vi "TARGET_856.vi"() -> ()   [LabVIEW 2018]
uses:
  <vilib>/Platform/TimedLoop/XDataNode/timing_clust.ctl
  <vilib>/Platform/TimedLoop/XDataNode/nitl_modes.ctl
  <vilib>/Platform/TimedLoop/XDataNode/wakeup.ctl
  <vilib>/rvi/eio/common/nirviEmuTemplateMethod_errors.vi
  <vilib>/rvi/Emulation/niFpgaGetClockAttributes.vi
  <vilib>/rvi/Emulation/niFpgaSctlEmulationGetInTimedLoop.vi
  <vilib>/rvi/Emulation/niFpgaEmulationReportErrorSimple.vi
  <vilib>/rvi/Emulation/niFpgaProcessEmulError.vi
  <vilib>/rvi/Emulation/niFpgaCriticalErrorInLSC.vi
  <vilib>/rvi/interface/RandomDataEmulation/niFpgaRandomDataHandleErrors.vi
  <vilib>/eio/EIONode/EIONode.xnode
  <vilib>/Platform/TimedLoop/XDataNode/XDataNode.xnode
  <vilib>/rvi/DataTransferAndStorage/Container/XNode/niFpgaContainer.xnode
  <vilib>/rvi/interface/RandomDataEmulation/nirviRandomDataFpgaReadWriteTemplate.vi
  <vilib>/Platform/TimedLoop/XDataNode/XDNodeRunTimeDep.lvlib
panel:
  out "READ":bool[](array[boolean])
  in  "Write Data":bool[](array[boolean])=[FALSE, FALSE, FALSE, FALSE, FALSE, FALSE, FALSE, FALSE, FALSE]
  in  "Enum":T1(ring)=enum."GREEN OFF"
  in  "Read(T)/Write(F)":bool
  in  "Command array":bool[](array[boolean])=[FALSE, FALSE, FALSE, FALSE, FALSE, FALSE, FALSE, FALSE, FALSE, FALSE, FALSE, FALSE, FALSE, FALSE, FALSE, FALSE, FALSE]
  in  "Конфигурация":bool
  in  "Остановка основного цикла":bool
  in  "Линейки":bool
  in  "Между кадрами":u8=1 caption="Между кадрами, мс"
  out "Элем.":u32
  out "Данные":u8
  in  "Направление бит":bool
  in  "CDS1_1":u8=2
  in  "CDS1_2":u8=4
  in  "CDS2_1":u8=5
  in  "CDS2_2":u8=7
  in  "ADC_1":u8=2
  in  "ADC_2":u8=7
  in  "RG_1":u8=1
  in  "RG_2":u8=2
  in  "PH21_1":u8=1
  in  "PH21_2":u8=6
  in  "PH11_1":u8=1
  in  "PH11_2":u8=6
  in  "HOR":u16=880
  in  "10":u8=10
  in  "LOW":u8=1
  in  "HIGH":u8=9
  in  "2017":u16=2017
  in  "PS1_2":u16=1809
  in  "PS1_1":u16=715
  in  "PS2_2":u16=1151
  in  "PS2_1":u16=496
  in  "PS3_2":u16=1589
  in  "PS3_1":u16=934
  in  "PS4_2":u16=1371
  in  "PS4_1":u16=277
  in  "Строка триггер":u16=50
  out "Какая строка":i32
  in  "Сколько строк?":i32=110
  in  "Кадр в FIFO":bool
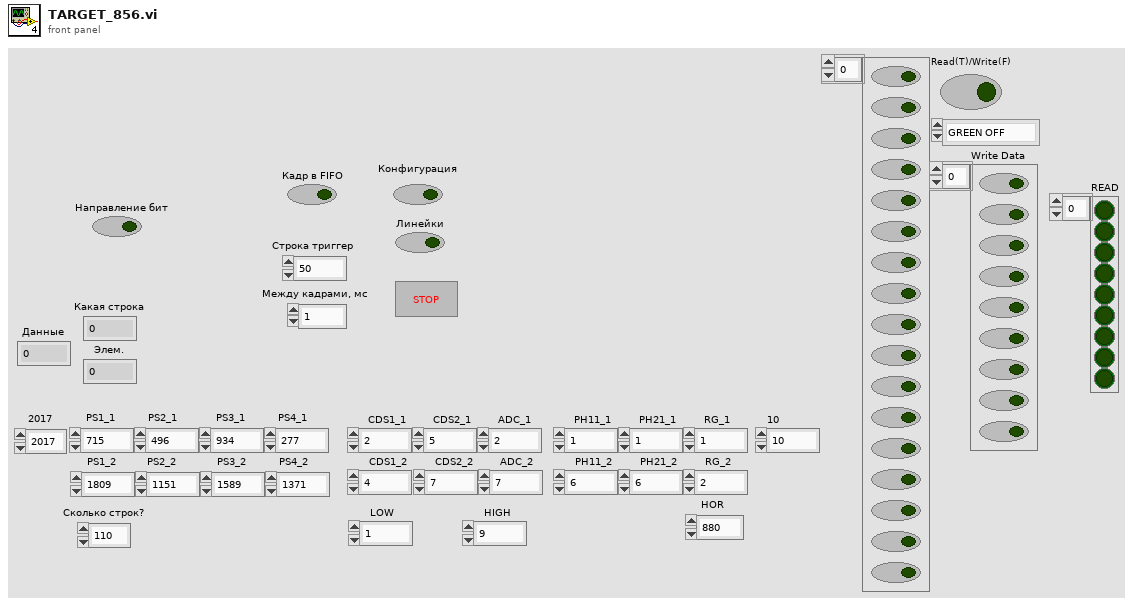
[diagram p1: front panel]
types:
  T1 = enum16{"Configuration", "MUX", "RED PGA", "GREEN PGA", "BLUE PGA", "RED OFF", "GREEN OFF", "BLUE OFF"}
  T2 = typedef "XDNodeRunTimeDep.lvlib/timing_clust.ctl" = cluster{"Expected End [f-1]":u64, "Actual End [f-1]":u64, "Finished Late? [f-1]":bool, "Expected End [i-1]":u64, "Actual End [i-1]":u64, "Finished Late? [i-1]":bool, "Expected Start [i]":u64, "Actual Start [i]":u64, "Expected Start [f]":u64, "Actual Start [f]":u64, "Source Name":string, "Structure Name":string, "Period":i64, "Deadline":i64, "Offset":i64, "Start":i64, "Priority":i32, "Timeout":i32, "Mode":T3, "Wakeup Reason":T4, "Error":errorcluster, "Source Type":string, "Secondary Source Type":string, "Global End Time":u64, "Global Start Time":u64, "Frame Duration":u64, "Iteration Duration":u64, "Assigned CPU":i32, "I/O Scan Engine Mode":u32}
  T3 = typedef "XDNodeRunTimeDep.lvlib/nitl_modes.ctl" = enum32{"No Change", "Process missed periods, maintain original phase", "Discard missed periods, maintain original phase", "Process missed periods, ignore original phase", "Discard missed periods, ignore original phase"}
  T4 = typedef "XDNodeRunTimeDep.lvlib/wakeup.ctl" = enum32{"Normal", "Aborted", "Asynchronous wakeup", "Timing source error", "Timed loop error", "Timeout"}
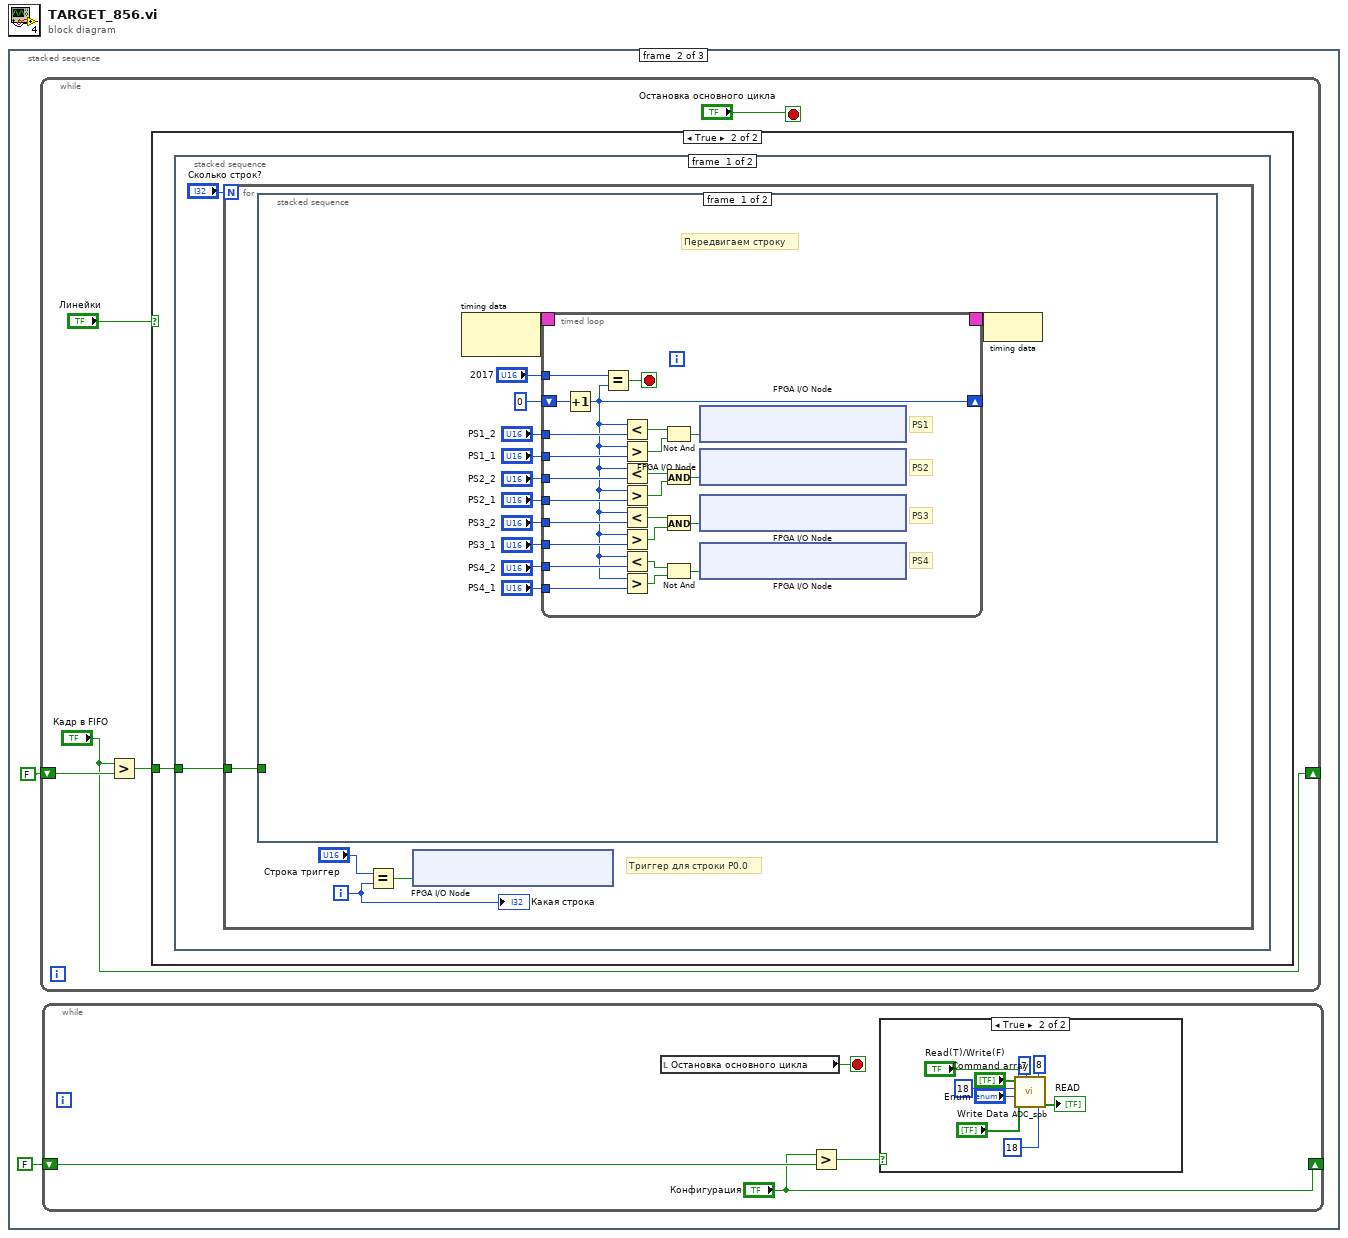
[diagram p0: block diagram]
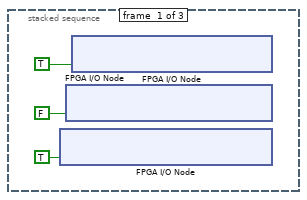
[diagram p2: hidden frame]
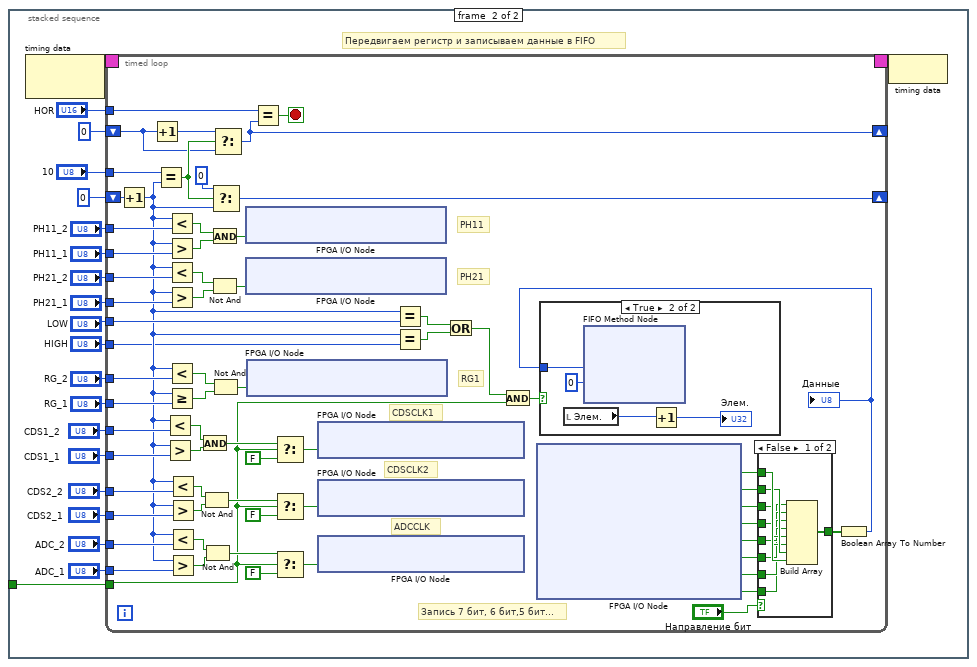
[diagram p4: hidden frame]
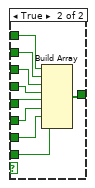
[diagram p5: hidden frame]
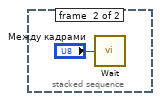
[diagram p7: hidden frame]
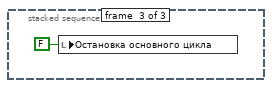
[diagram p9: hidden frame]
diagram:
  n1 = stacked-sequence {
    frame #0 {
      n2 = xnode "FPGA I/O Node"("IO Module\\DDCA_DIO16-23_WE"=TRUE) -> ()  [unwired: 1 in, 1 out]
      n3 = xnode "FPGA I/O Node"("IO Module\\DDCA_DIO8-15_WE"=FALSE) -> ()  [unwired: 1 in, 1 out]
      n4 = xnode "FPGA I/O Node"("IO Module\\DDCA_DIO0-7_WE"=TRUE) -> ()  [unwired: 1 in, 1 out]
    }
    frame #1 {
      n5 = while {
        shift-right: ["Кадр в FIFO"] -> _
        shift-left: FALSE ("Кадр в память") -> [w8]
        stop <- "Остановка основного цикла" stop-if-true
        n6 = Greater?(x="Кадр в FIFO", y=w8) -> (0:w6:bool)
        n7 = case shown="True" "Линейки" {
          tunnel: w6 -> [_ w11]
          frame False {
          }
          frame True {
            n8 = stacked-sequence {
              tunnel: w11 -> [w12 _]
              frame #0 {
                n9 = for {
                  N: "Сколько строк?" -> [_]
                  tunnel: w12 -> [w17]
                  i -> [w15]
                  # "Триггер для строки Р0.0"
                  n10 = stacked-sequence {
                    tunnel: w17 -> [_ w76]
                    frame #0 {
                      # "Передвигаем строку"
                      n11 = node-c288() -> (w29:T2)  [unwired: 1 in]
                      n12 = timed-loop {
                        timing: w29 -> [_]
                        timing-out: [_] -> w28
                        tunnel: "2017" -> [w52]
                        shift-right: [w30] -> _
                        shift-left: u16 0 -> [w53]
                        tunnel: "PS1_2" -> [w46]
                        tunnel: "PS1_1" -> [w45]
                        tunnel: "PS2_2" -> [w44]
                        tunnel: "PS2_1" -> [w43]
                        tunnel: "PS3_2" -> [w42]
                        tunnel: "PS3_1" -> [w41]
                        tunnel: "PS4_2" -> [w40]
                        tunnel: "PS4_1" -> [w39]
                        stop <- w51 stop-if-true
                        # "PS4"
                        # "PS3"
                        # "PS2"
                        # "PS1"
                        n13 = Increment(x=w53) -> (x+1=w30:u16)
                        n14 = Equal?(x=w52, y=w30) -> (x = y?=w51:bool)
                        n15 = Less?(x=w30, y=w46) -> (x < y?=w38:bool)
                        n16 = Greater?(x=w30, y=w45) -> (0:w37:bool)
                        n17 = Less?(x=w30, y=w44) -> (x < y?=w36:bool)
                        n18 = Greater?(x=w30, y=w43) -> (0:w35:bool)
                        n19 = Less?(x=w30, y=w42) -> (x < y?=w34:bool)
                        n20 = Greater?(x=w30, y=w41) -> (0:w33:bool)
                        n21 = Less?(x=w30, y=w40) -> (x < y?=w32:bool)
                        n22 = Greater?(x=w30, y=w39) -> (0:w31:bool)
                        n23 = Not And(1:w37, 2:w38) -> (0:w50:bool)
                        n24 = And(x=w36, y=w35) -> (x .and. y?=w49:bool)
                        n25 = And(x=w34, y=w33) -> (x .and. y?=w48:bool)
                        n26 = Not And(1:w31, 2:w32) -> (0:w47:bool)
                        n27 = xnode "FPGA I/O Node"("IO Module\\DDCA_DIO22_Write"=w50) -> ()  [unwired: 1 in, 1 out]
                        n28 = xnode "FPGA I/O Node"("IO Module\\DDCA_DIO21_Write"=w49) -> ()  [unwired: 1 in, 1 out]
                        n29 = xnode "FPGA I/O Node"("IO Module\\DDCA_DIO23_Write"=w48) -> ()  [unwired: 1 in, 1 out]
                        n30 = xnode "FPGA I/O Node"("IO Module\\DDCA_DIO20_Write"=w47) -> ()  [unwired: 1 in, 1 out]
                      }
                      n31 = node-c288(w28) -> ()
                    }
                    frame #1 {
                      # "Передвигаем регистр и записываем данные в FIFO"
                      n32 = node-c288() -> (w78:T2)  [unwired: 1 in]
                      n33 = timed-loop {
                        timing: w78 -> [_]
                        timing-out: [_] -> w77
                        tunnel: w76 -> [w118]
                        tunnel: "ADC_1" -> [w113]
                        tunnel: "ADC_2" -> [w112]
                        tunnel: "CDS2_1" -> [w111]
                        tunnel: "CDS2_2" -> [w110]
                        tunnel: "CDS1_1" -> [w109]
                        tunnel: "CDS1_2" -> [w108]
                        tunnel: "RG_1" -> [w107]
                        tunnel: "RG_2" -> [w106]
                        tunnel: "PH21_1" -> [w105]
                        tunnel: "PH21_2" -> [w104]
                        tunnel: "PH11_1" -> [w103]
                        tunnel: "PH11_2" -> [w102]
                        tunnel: "HOR" -> [w97]
                        shift-right: [w101] -> _
                        shift-left: u8 0 -> [w116]
                        tunnel: "10" -> [w114]
                        shift-right: [w96] -> _
                        shift-left: u16 0 ("Numeric") -> [w98]
                        tunnel: "LOW" -> [w91]
                        tunnel: "HIGH" -> [w89]
                        stop <- w95 stop-if-true
                        # "Запись 7 бит, 6 бит,5 бит..."
                        # "RG1"
                        # "PH21"
                        # "PH11"
                        # "ADCCLK"
                        # "CDSCLK2"
                        # "CDSCLK1"
                        n34 = Increment(x=w116) -> (x+1=w90:u8)
                        n35 = Increment(x=w98) -> (x+1=w99:u16)
                        n36 = Equal?(x=w114, y=w90) -> (x = y?=w100:bool)
                        n37 = Less?(x=w90, y=w108) -> (x < y?=w134:bool)
                        n38 = Greater?(x=w90, y=w109) -> (0:w133:bool)
                        n39 = Less?(x=w90, y=w102) -> (x < y?=w125:bool)
                        n40 = Greater?(x=w90, y=w103) -> (0:w124:bool)
                        n41 = Less?(x=w90, y=w104) -> (x < y?=w123:bool)
                        n42 = Greater?(x=w90, y=w105) -> (0:w122:bool)
                        n43 = Less?(x=w90, y=w106) -> (x < y?=w121:bool)
                        n44 = Greater Or Equal?(x=w90, y=w107) -> (x >= y?=w120:bool)
                        n45 = Less?(x=w90, y=w110) -> (x < y?=w131:bool)
                        n46 = Greater?(x=w90, y=w111) -> (0:w132:bool)
                        n47 = Less?(x=w90, y=w112) -> (x < y?=w130:bool)
                        n48 = Greater?(x=w90, y=w113) -> (0:w129:bool)
                        n49 = And(x=w134, y=w133) -> (x .and. y?=w137:bool)
                        n50 = Not And(1:w132, 2:w131) -> (0:w138:bool)
                        n51 = Not And(1:w129, 2:w130) -> (0:w139:bool)
                        n52 = And(x=w125, y=w124) -> (x .and. y?=w128:bool)
                        n53 = Not And(1:w122, 2:w123) -> (0:w127:bool)
                        n54 = Select(t=u8 0, s=w100, f=w90) -> (s? t:f=w101:u8)
                        n55 = Not And(1:w120, 2:w121) -> (0:w126:bool)
                        n56 = Select(t=w99, s=w100, f=w98) -> (s? t:f=w96:u16)
                        n57 = xnode "FPGA I/O Node"("IO Module\\DDCA_DIO4_Write"=w128) -> ()  [unwired: 1 in, 1 out]
                        n58 = xnode "FPGA I/O Node"("IO Module\\DDCA_DIO3_Write"=w127) -> ()  [unwired: 1 in, 1 out]
                        n59 = xnode "FPGA I/O Node"("IO Module\\DDCA_DIO2_Write"=w126) -> ()  [unwired: 1 in, 1 out]
                        n60 = Equal?(x=w97, y=w96) -> (x = y?=w95:bool)
                        n61 = Select(t=w137, s=w118, f=FALSE) -> (s? t:f=w135:bool)
                        n62 = Select(t=w138, s=w118, f=FALSE) -> (s? t:f=w136:bool)
                        n63 = Select(t=w139, s=w118, f=FALSE) -> (s? t:f=w143:bool)
                        n64 = xnode "FPGA I/O Node"("IO Module\\DDCA_DIO18_Write"=w135) -> ()  [unwired: 1 in, 1 out]
                        n65 = xnode "FPGA I/O Node"("IO Module\\DDCA_DIO17_Write"=w136) -> ()  [unwired: 1 in, 1 out]
                        n66 = xnode "FPGA I/O Node"("IO Module\\DDCA_DIO16_Write"=w143) -> ()  [unwired: 1 in, 1 out]
                        n67 = Equal?(x=w90, y=w91) -> (x = y?=w94:bool)
                        n68 = Equal?(x=w90, y=w89) -> (x = y?=w93:bool)
                        n69 = Or(x=w94, y=w93) -> (x .or. y?=w117:bool)
                        n70 = And(x=w117, y=w118) -> (x .and. y?=w119:bool)
                        n71 = xnode "FPGA I/O Node"() -> ("IO Module\\DDCA_DIO8_Read"=w88:bool, "IO Module\\DDCA_DIO9_Read"=w87:bool, "IO Module\\DDCA_DIO10_Read"=w86:bool, "IO Module\\DDCA_DIO11_Read"=w84:bool, "IO Module\\DDCA_DIO12_Read"=w83:bool, "IO Module\\DDCA_DIO13_Read"=w82:bool, "IO Module\\DDCA_DIO14_Read"=w81:bool, "IO Module\\DDCA_DIO15_Read"=w80:bool)  [unwired: 8 in, 8 out]
                        n72 = case shown="False" "Направление бит" {
                          tunnel: w88 -> [w151 w161]
                          tunnel: w87 -> [w150 w160]
                          tunnel: w86 -> [w149 w159]
                          tunnel: w84 -> [w148 w158]
                          tunnel: w83 -> [w147 w157]
                          tunnel: w82 -> [w146 w156]
                          tunnel: w81 -> [w145 w155]
                          tunnel: w80 -> [w144 w154]
                          tunnel: [w152 w153] -> w79
                          frame False {
                            n73 = Build Array(w144, w145, w146, w147, w148, w149, w150, w151) -> (w152:bool[])
                          }
                          frame True {
                            n74 = Build Array(w161, w160, w159, w158, w157, w156, w155, w154) -> (w153:bool[])
                          }
                        }
                        n75 = Boolean Array To Number(Boolean array=w79) -> (number=w92:u8)
                        "Данные" <- w92
                        n76 = case shown="True" w119 {
                          tunnel: w92 -> [_ w164]
                          frame False {
                          }
                          frame True {
                            n77 = local read "Элем."() -> (w163:u32)
                            n78 = xnode ("FIFO Method Node")("Element"=w164, "Timeout"=0) -> ()  [unwired: 1 in, 2 out]
                            n79 = Increment(x=w163) -> (x+1=→"Элем.":u32)
                          }
                        }
                      }
                      n80 = node-c288(w77) -> ()
                    }
                  }
                  n81 = Equal?(x="Строка триггер", y=w15) -> (x = y?=w14:bool)
                  n82 = xnode "FPGA I/O Node"("IO Module\\DDCA_DIO0_Write"=w14) -> ()  [unwired: 1 in, 1 out]
                  "Какая строка" <- w15
                }
              }
              frame #1 {
                n83 = call "Wait"("Count(mSec)"="Между кадрами") -> ()  [unwired: 1 out]
              }
            }
          }
        }
      }
      n84 = while {
        shift-right: ["Конфигурация"] -> _
        shift-left: FALSE ("Конфигурация") -> [w173]
        stop <- w174 stop-if-true
        n85 = local read "Остановка основного цикла"() -> (w174:bool)
        n86 = Greater?(x="Конфигурация", y=w173) -> (0:w171:bool)
        n87 = case shown="True" w171 {
          frame False {
          }
          frame True {
            n88 = call "ADC_spb.vi"(1:"18_1"=i8 18 ("18_1"), 2:"18_1"=i8 18 ("18_1"), "8"=i8 8, "7"=i8 7, "Write Data"="Write Data", "Enum"="Enum", "Read(T)/Write(F)"="Read(T)/Write(F)", "Command array"="Command array") -> ("READ"=→"READ":bool[])
          }
        }
      }
    }
    frame #2 {
      n89 = local write "Остановка основного цикла"(FALSE ("Остановка основного цикла")) -> ()
    }
  }
